vi "Constructor by Ctrl Label.vi"(8 "error in (no error)":errorcluster, 9 "Database (use member data)":refnum<class "Database.lvclass">, 10 "Ctl Refnum":refnum<vi>, 11 "Field in":refnum<class "Field.lvclass">) -> (0 "error out":errorcluster, 3 "Field out":refnum<class "Field.lvclass">)   [LabVIEW 2020, in "Field.lvlib" / "Field.lvclass"]
uses:
  Field.lvclass
  Database/Database Class/Database.lvclass
  Field.lvclass/Field.ctl
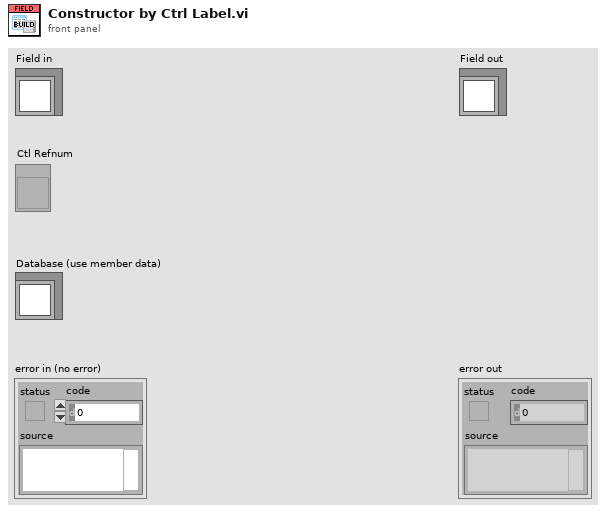
[diagram p1: front panel]
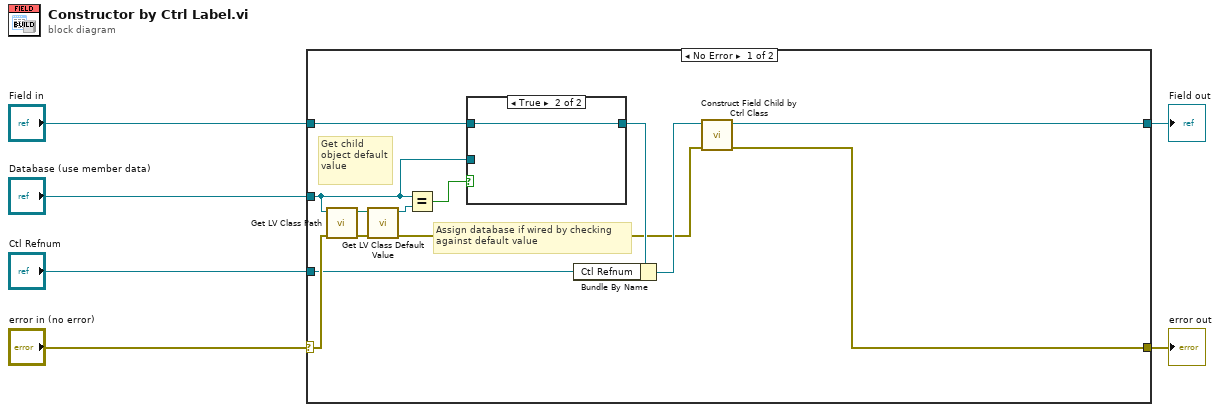
[diagram p0: block diagram]
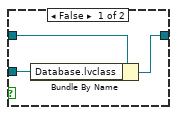
[diagram p2: hidden frame]
diagram:
  n1 = case shown="No Error" "error in (no error)" {
    selector: "error in (no error)" -> [w13 w25]
    tunnel: [w7 w25] -> w5
    tunnel: [w9 w24] -> w3
    tunnel: "Field in" -> [w14 w24]
    tunnel: "Database (use member data)" -> [w15 _]
    tunnel: "Ctl Refnum" -> [w11 _]
    frame No Error {
      # "Get child object default value"
      # "Assign database if wired by checking\nagainst default value"
      n2 = call <vilib>:"Get LV Class Path.vi"("error in (no error)"=w13, "object"=w15) -> ("error out"=w18:errorcluster, "class path"=w19:path)  [unwired: 8 in]
      n3 = call <vilib>:"Get LV Class Default Value.vi"("error in (no error)"=w18, "class path"=w19) -> ("error out"=w8:errorcluster, "object"=w17:refnum<class>)  [unwired: 8 in]
      n4 = Equal?(x=w15, y=w17) -> (x = y?=w16:bool)
      n5 = case shown="True" w16 {
        tunnel: w15 -> [w21 _]
        tunnel: w14 -> [w22 w23]
        tunnel: [w20 w23] -> w12
        frame False {
          n6 = Bundle By Name(cluster=w22, "Database.lvclass"=w21) -> (w20:refnum<class "Field.lvclass">)
        }
        frame True {
        }
      }
      n7 = Bundle By Name(cluster=w12, "Ctl Refnum"=w11) -> (w10:refnum<class "Field.lvclass">)
      n8 = call "Construct Field Child by Ctrl Class.vi"("error in (no error)"=w8, "Field in"=w10) -> ("error out"=w7:errorcluster, "Field out"=w9:refnum<class "Field.lvclass">)  [unwired: 8 in]
    }
    frame Error {
    }
  }
  "error out" <- w5
  "Field out" <- w3
